vi "设置模块队列名.vi"() -> (2 "Msg":string)   [LabVIEW 2016, in "斯坦道总磷总氮.lvlib"]
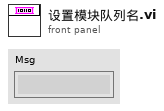
[diagram p1: front panel]
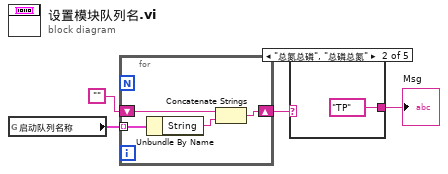
[diagram p0: block diagram]
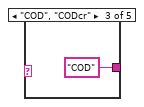
[diagram p3: hidden frame]
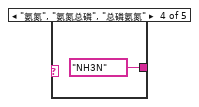
[diagram p4: hidden frame]
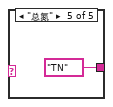
[diagram p5: hidden frame]
diagram:
  n1 = global read "总磷总氮断电保存全局变量.vi" "启动队列名称"() -> (w2:cluster{"String":string, "Value":u16}[])
  n2 = for {
    tunnel: w2 -> [w8] mode=indexing
    shift-right: [w7] -> w1
    shift-left: "" -> [w5]
    n3 = Unbundle By Name(w8) -> ("String"=w6:string)
    n4 = Concatenate Strings(w5, w6) -> (w7:string)
  }
  n5 = case shown="\"总氮总磷\", \"总磷总氮\"" w1 {
    selector: w1 -> [w9 _ _ _ _]
    tunnel: [w9 "TP" ("队列名") "COD" ("队列名") "NH3N" ("队列名") "TN" ("队列名")] -> w4
    frame Default {
    }
    frame "总氮总磷", "总磷总氮" {
    }
    frame "COD", "CODcr" {
    }
    frame "氨氮", "氨氮总磷", "总磷氨氮" {
    }
    frame "总氮" {
    }
  }
  "Msg" <- w4
